vi "Check Name.vi"(7 "Existing PIDs":string[](array[string]), 8 "error in (no error)":errorcluster, 10 "ID":refnum<vi>, 11 "Name":refnum<vi>) -> (0 "error out":errorcluster, 2 "String":string, 3 "Boolean":bool)   [LabVIEW 2015, in "Diagnostics Addon System Explorer.lvlib"]
uses:
  Diagnostics Addon System Explorer.lvlib
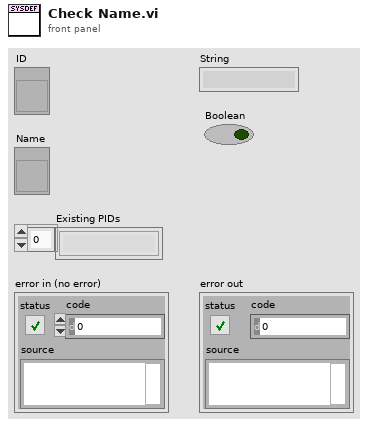
[diagram p1: front panel]
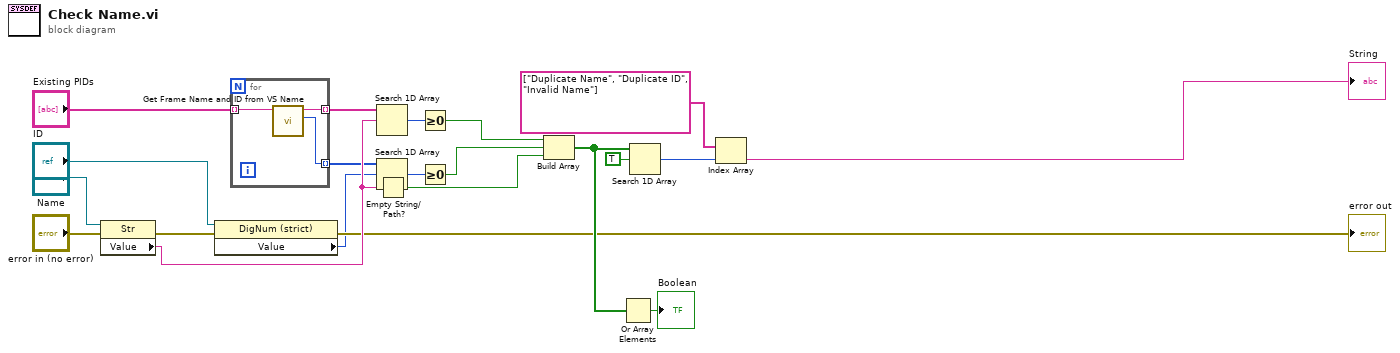
[diagram p0: block diagram]
diagram:
  n1 = property class="Str"(reference="Name", error in="error in (no error)") -> (error out=w2:errorcluster, "Value"=w12:string)  [unwired: 1 out]
  n2 = property class="DigNum (strict)"(reference="ID", error in=w2) -> (error out=→"error out":errorcluster, "Value"=w7:u16)  [unwired: 1 out]
  n3 = for {
    tunnel: "Existing PIDs" -> [w24] mode=indexing
    tunnel: [w23] -> w6 mode=indexing
    tunnel: [w22] -> w8 mode=indexing
    n4 = call "Get Frame Name and ID from VS Name.vi"("VS PID Name"=w24) -> ("ID"=w23:u16, "PID Name"=w22:string)  [unwired: 9 in]
  }
  n5 = Search 1D Array(1D array=w8, element=w12) -> (index of element=w11:i32)  [unwired: 1 in]
  n6 = Search 1D Array(1D array=w6, element=w7) -> (index of element=w10:i32)  [unwired: 1 in]
  n7 = Empty String/Path?(string/path=w12) -> (empty?=w20:bool)
  n8 = Greater Or Equal To 0?(x=w11) -> (x >= 0?=w18:bool)
  n9 = Greater Or Equal To 0?(x=w10) -> (x >= 0?=w19:bool)
  n10 = Build Array(w18, w19, w20) -> (w14:bool[])
  n11 = Or Array Elements(Boolean array=w14) -> (logical OR=→"Boolean":bool)
  n12 = Search 1D Array(1D array=w14, element=TRUE) -> (index of element=w16:i32)  [unwired: 1 in]
  n13 = Index Array(array=string[] ["Duplicate Name", "Duplicate ID", "Invalid Name"], index=w16) -> (element=→"String":string)
